vi "panStamp_processPacket.vi"(8 "error in":errorcluster, 9 "packet_in":string="703100000327010100F245464748494A4B4C4D4E4F505152535455565758595A", 11 "Status In":T1) -> (0 "error out":errorcluster, 1 "formatted text out":string, 3 "Status Out":T1, 4 "update":bool, 5 "RSSI":dbl(slide))   [LabVIEW 2014]
uses:
  <vilib>/imath/engines/lvmath/Plug In/_Char/NIMS_CH_character datatype.ctl
  <vilib>/imath/engines/lvmath2/RunTimeEngine/BuiltInFunctions/length/NIMS_length(GV).vi
  <instcachedir>/0/NIMS_length(GV)_08A3D13377FD4E4B96F5795FBF3698FA.lvgen/NIMS_length(GV)_08A3D13377FD4E4B96F5795FBF3698FA_003.vi
  <vilib>/imath/engines/lvmath2/RunTimeEngine/IndexRead/NIMS V(S).vi
  <instcachedir>/0/NIMS V(S)_0488751826AF41519A22953C041130DC.lvgen/NIMS V(S)_0488751826AF41519A22953C041130DC_003.vi
  <vilib>/imathl/engines/lvmath/Functions/Error Handling/Create Error.vi
  <vilib>/imath/engines/lvmath2/RunTimeEngine/ErrorHandling/NIMS_Create Error From Enums.vi
  <vilib>/imath/engines/lvmath2/RunTimeEngine/VariableToken/NIMS_VariableToken_CondDefined.vi
  <instcachedir>/0/NIMS_VariableToken_CondDefined_EE8DD211A89249938CE6537267F5C9B3.lvgen/NIMS_VariableToken_CondDefined_EE8DD211A89249938CE6537267F5C9B3_004.vi
  <instcachedir>/0/NIMS_VariableToken_CondDefined_EE8DD211A89249938CE6537267F5C9B3.lvgen/NIMS_VariableToken_CondDefined_EE8DD211A89249938CE6537267F5C9B3_005.vi
  <instcachedir>/0/NIMS_VariableToken_CondDefined_EE8DD211A89249938CE6537267F5C9B3.lvgen/NIMS_VariableToken_CondDefined_EE8DD211A89249938CE6537267F5C9B3_006.vi
  <vilib>/imath/engines/lvmath/Plug In/_Char/NIMS_CH_Character RV to String.vi
  <vilib>/imath/engines/lvmath/Functions/Error Handling/MergeErrorsWrapper.vi
  <vilib>/imath/engines/lvmath2/RunTimeEngine/NodeEndStatement/NIMS_NodeEndStatement_Output.vi
  <instcachedir>/0/NIMS_NodeEndStatement_Output_53EC0D466D134D7ABD903AC30B43404B.lvgen/NIMS_NodeEndStatement_Output_53EC0D466D134D7ABD903AC30B43404B_001.vi
  <instcachedir>/0/NIMS_NodeEndStatement_Output_53EC0D466D134D7ABD903AC30B43404B.lvgen/NIMS_NodeEndStatement_Output_53EC0D466D134D7ABD903AC30B43404B_014.vi
  <instcachedir>/0/NIMS_NodeEndStatement_Output_53EC0D466D134D7ABD903AC30B43404B.lvgen/NIMS_NodeEndStatement_Output_53EC0D466D134D7ABD903AC30B43404B_009.vi
  <instcachedir>/0/NIMS_NodeEndStatement_Output_53EC0D466D134D7ABD903AC30B43404B.lvgen/NIMS_NodeEndStatement_Output_53EC0D466D134D7ABD903AC30B43404B_012.vi
  <instcachedir>/0/NIMS_NodeEndStatement_Output_53EC0D466D134D7ABD903AC30B43404B.lvgen/NIMS_NodeEndStatement_Output_53EC0D466D134D7ABD903AC30B43404B_011.vi
  <vilib>/imath/engines/lvmath2/RunTimeEngine/ErrorHandling/NIMS_Finalize Error.vi
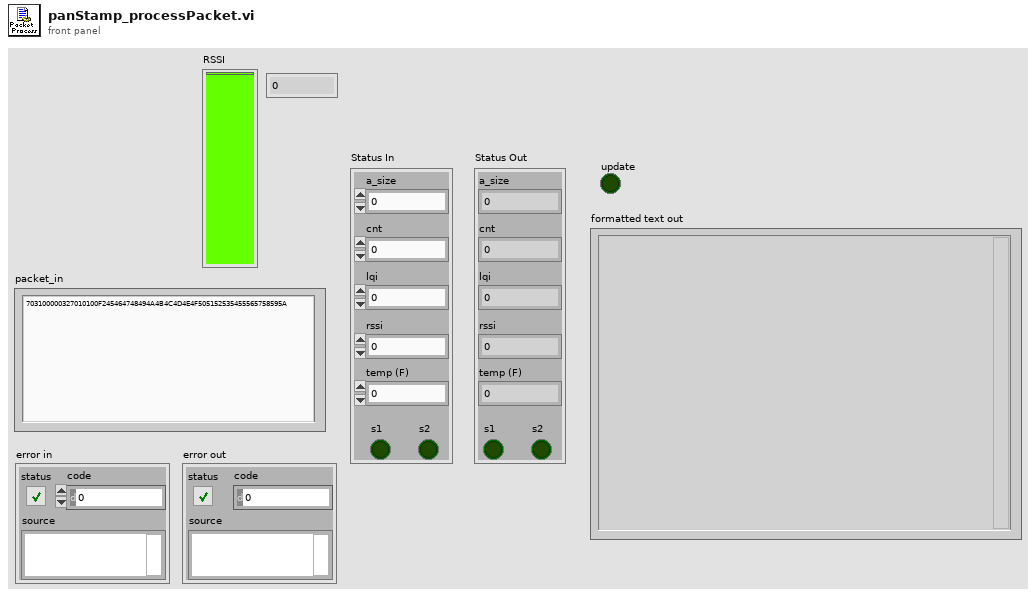
[diagram p1: front panel]
types:
  T1 = cluster{"rssi":dbl, "a_size":i32, "lqi":u8, "cnt":dbl, "s1":bool, "s2":bool, "temp (F)":dbl}
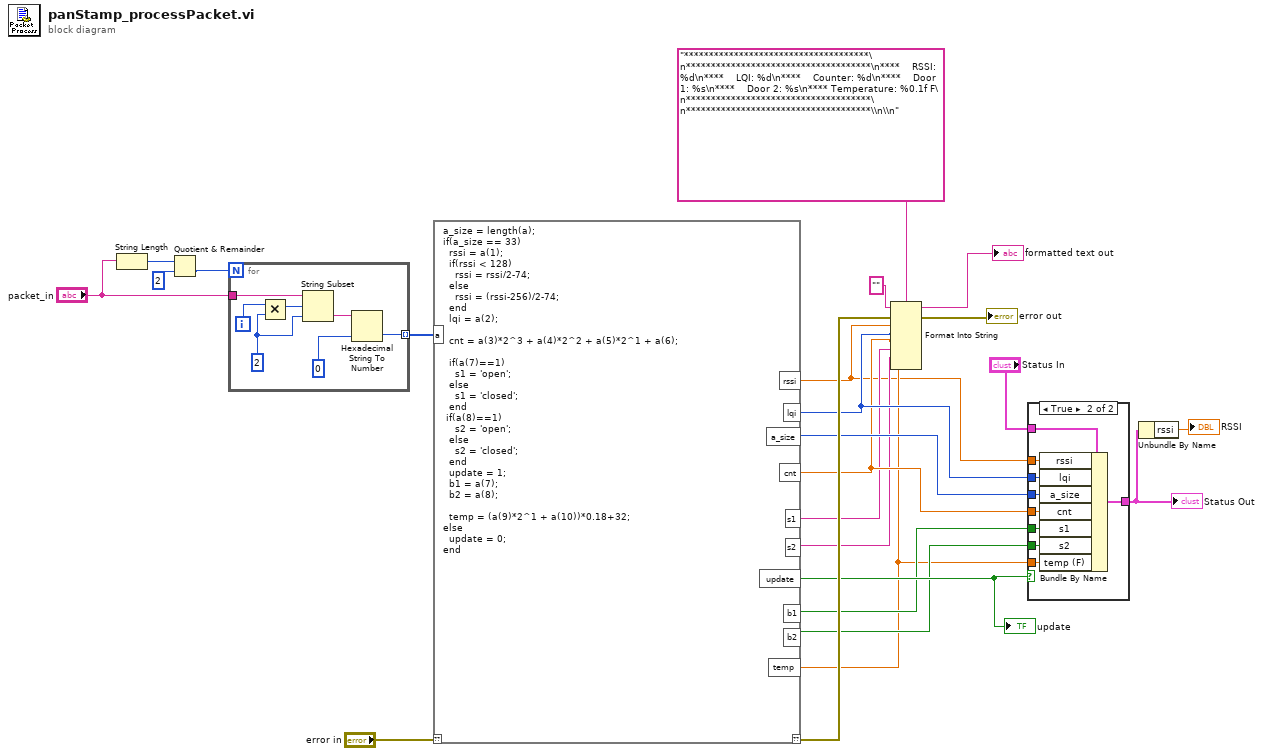
[diagram p0: block diagram]
diagram:
  n1 = String Length(string="packet_in") -> (length=w24:i32)
  n2 = Quotient & Remainder(x=w24, y=2) -> (floor(x/y)=w15:i32)  [unwired: 1 out]
  n3 = for {
    N: w15 -> [_]
    tunnel: "packet_in" -> [w30]
    tunnel: [w26] -> w22 mode=indexing
    i -> [w29]
    w25 = 2
    n4 = Multiply(x=w29, y=w25) -> (x*y=w31:i32)
    n5 = String Subset(string=w30, offset (0)=w31, length (rest)=w25) -> (substring=w28:string)
    n6 = Hexadecimal String To Number(string=w28, default (0uL)=u8 0) -> (number=w26:u8)  [unwired: 1 in, 1 out]
  }
  n7 = mathscript code="a_size = length(a);\nif(a_size == 33)\n  rssi = a(1);\n  if(rssi < 128)\n    rssi = rssi/2-74;\n  else\n    rssi = (rssi-256)/2-74;\n  end\n  lqi = a(2);\n\n  cnt = a(3)*2^3 + a(4)*2^2 + a(5)*2^1 + a(6);\n\n  if(a(7)==1)\n    s1 = 'open';\n  else\n    s1 = 'closed';\n  end\n if(a(8)==1)\n    s2 = 'open';\n  else\n    s2 = 'closed';\n  end\n  update = 1;\n  b1 = a(7);\n  b2 = a(8);\n\n  temp = (a(9)*2^1 + a(10))*0.18+32;\nelse\n  update = 0;\nend"("??"="error in", "a"=w22) -> ("??"=w18:errorcluster, "rssi"=w3:dbl, "a_size"=w13:i32, "lqi"=w14:u8, "cnt"=w12:dbl, "s1"=w9:string, "s2"=w8:string, "update"=w11:bool, "b1"=w7:bool, "b2"=w6:bool, "temp"=w4:dbl)
  "update" <- w11
  n8 = Format Into String(format string="*************************************\n*************************************\n****    RSSI: %d\n****    LQI: %d\n****    Counter: %d\n****    Door 1: %s\n****    Door 2: %s\n**** Temperature: %0.1f F\n*************************************\n*************************************\\n\\n", initial string="", error in=w18, w3, w14, w12, w9, w8, w4) -> (resulting string=→"formatted text out":string, error out=→"error out":errorcluster)
  n9 = case shown="True" w11 {
    tunnel: w3 -> [_ w41]
    tunnel: w14 -> [_ w40]
    tunnel: w13 -> [_ w39]
    tunnel: w12 -> [_ w38]
    tunnel: w7 -> [_ w37]
    tunnel: [w32 w36] -> w2
    tunnel: "Status In" -> [w32 w35]
    tunnel: w6 -> [_ w34]
    tunnel: w4 -> [_ w33]
    frame False {
    }
    frame True {
      n10 = Bundle By Name(cluster=w35, "rssi"=w41, "lqi"=w40, "a_size"=w39, "cnt"=w38, "s1"=w37, "s2"=w34, "temp (F)"=w33) -> (w36:T1)
    }
  }
  "Status Out" <- w2
  n11 = Unbundle By Name(w2) -> ("rssi"=→"RSSI":dbl)
